vi "Read Power Impl.vi"(8 "error in (no error)":errorcluster, 11 "Thorlabs Power Meter in":refnum<class "Thorlabs Power Meter.lvclass">) -> (0 "error out":errorcluster, 2 "Raw Device Reading (W)":dbl=-1.0 caption="Power", 3 "Thorlabs Power Meter out":refnum<class "Thorlabs Power Meter.lvclass">)   [LabVIEW 2023, in "Thorlabs Power Meter.lvlib" / "Thorlabs Power Meter.lvclass"]
uses:
  Thorlabs Power Meter.lvclass
  Thorlabs Power Meter.lvclass/Thorlabs Power Meter.ctl
  Thorlabs Power Meter.lvlib
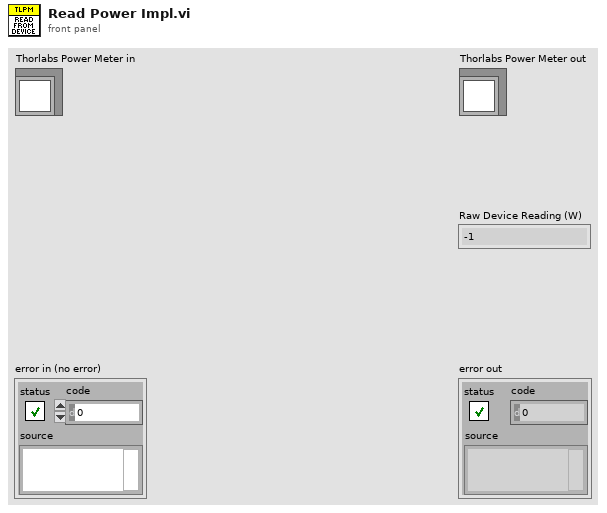
[diagram p1: front panel]
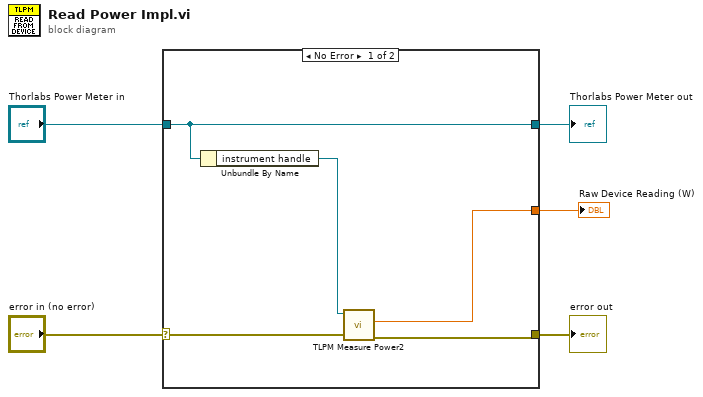
[diagram p0: block diagram]
diagram:
  n1 = case shown="No Error" "error in (no error)" {
    selector: "error in (no error)" -> [w9 w12]
    tunnel: [w7 w12] -> w4
    tunnel: "Thorlabs Power Meter in" -> [w10 w11]
    tunnel: [w10 w11] -> w2
    tunnel: [w6 _] -> w1
    frame No Error {
      n2 = Unbundle By Name(w10) -> ("instrument handle"=w8:refnum<visa-resource-name>)
      n3 = call "TLPM Measure Power2.vi"("error in (no error)"=w9, "instrument handle"=w8) -> ("error out"=w7:errorcluster, "Power"=w6:dbl)  [unwired: 7 in, 1 out]
    }
    frame Error {
    }
  }
  "error out" <- w4
  "Thorlabs Power Meter out" <- w2
  "Raw Device Reading (W)" <- w1
